vi "Initialization VI.vi"(8 "error in (no error)":errorcluster, 10 "Custom XML":string, 11 "Device Item Ref in":T1 format="%.0x") -> (0 "error out":errorcluster, 3 "Device Item Ref out":T1 format="%.0x")   [LabVIEW 2016, in "PXImc Custom Device System Explorer.lvlib"]
uses:
  PXImc Custom Device System Explorer.lvlib
  <vilib>/NI Veristand/Custom Device API/Custom Device Item Ref.ctl
  <vilib>/NI/NI VeriStand Custom Device Import and Export Tool/ImportExport.lvlib
  <vilib>/NI VeriStand/Custom Device API/Custom Device API.lvlib
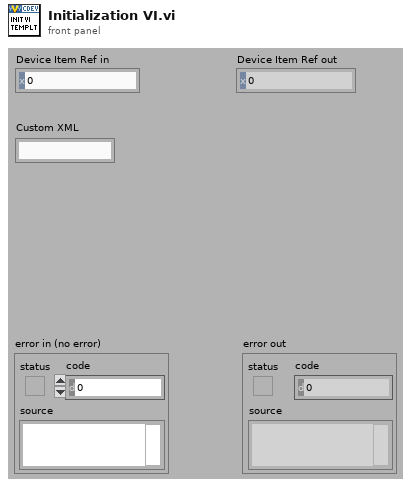
[diagram p1: front panel]
types:
  T1 = typedef "Custom Device API.lvlib/Custom Device Item Ref.ctl" = u64
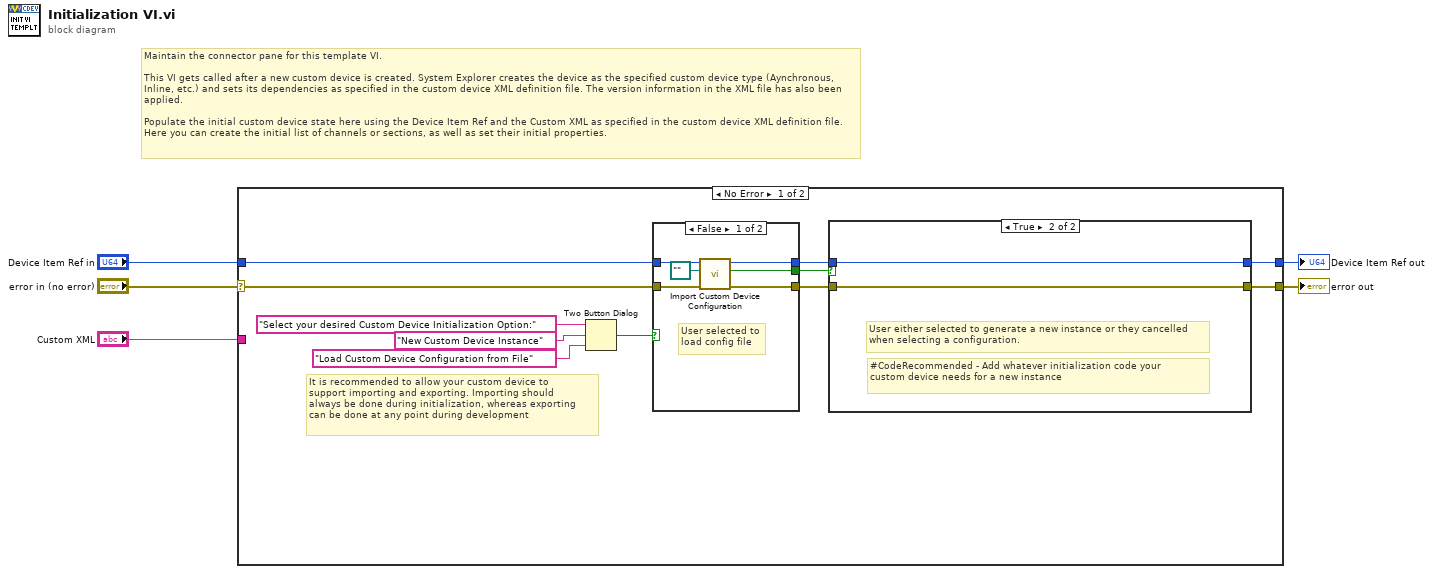
[diagram p0: block diagram]
diagram:
  # "Maintain the connector pane for this template VI.\n\nThis VI gets called after a new custom device is created. System Explorer creates the device as the specified custom device type (Aynchronous, Inline, etc.) and sets its dependencies as specified in the custom device XML definition file. The version information in the XML file has also been applied.\n\nPopulate the initial custom device state here using the Device Item Ref and the Custom XML as specified in the custom device XML definition file. Here you can create the initial list of channels or sections, as well as set their initial properties."
  n1 = case shown="No Error" "error in (no error)" {
    selector: "error in (no error)" -> [w11 w31]
    tunnel: [w7 w31] -> w5
    tunnel: [w6 w30] -> w3
    tunnel: "Device Item Ref in" -> [w12 w30]
    tunnel: "Custom XML" -> [_ _]
    frame No Error {
      # "It is recommended to allow your custom device to\nsupport importing and exporting. Importing should\nalways be done during initialization, whereas exporting\ncan be done at any point during development"
      n2 = Two Button Dialog(message="Select your desired Custom Device Initialization Option:", 1:"Load Custom Device Configuration from File" ("F button name (\"Cancel\")"), 2:"New Custom Device Instance" ("T button name (\"OK\")")) -> (T button?=w13:bool)
      n3 = case shown="False" w13 {
        selector: w13 -> [_ w27]
        tunnel: w12 -> [w26 w29]
        tunnel: [w25 w29] -> w10
        tunnel: w11 -> [w23 w28]
        tunnel: [w22 w28] -> w8
        tunnel: [w21 w27] -> w9
        frame False {
          # "User selected to\nload config file"
          n4 = call <vilib>:"Import Custom Device Configuration.vi"("error in (no error)"=w23, "Path"=path "", "NodeID"=w26) -> ("error out"=w22:errorcluster, "cancelled"=w21:bool, "NodeID out"=w25:u64)  [unwired: 6 in]
        }
        frame True {
          # "User selected new\ncustom device. Do\nnothing in this case\nand handle new\ngeneration in the\nnext case structure"
        }
      }
      n5 = case shown="True" w9 {
        tunnel: w10 -> [w18 w19]
        tunnel: w8 -> [w17 w20]
        tunnel: [w17 w20] -> w7
        tunnel: [w18 w19] -> w6
        frame False {
          # "User selected to import from configuration and didn't cancel import"
        }
        frame True {
          # "#CodeRecommended - Add whatever initialization code your\ncustom device needs for a new instance"
          # "User either selected to generate a new instance or they cancelled\nwhen selecting a configuration."
        }
      }
    }
    frame Error {
    }
  }
  "error out" <- w5
  "Device Item Ref out" <- w3
